vi "Output BPM.vi"(4 "error in (no error)":errorcluster, 7 "BPM (input)":dbl) -> (0 "error out":errorcluster, 3 "BPM (output)":string)   [LabVIEW 2012]
doc: "Takes the BPM input and outputs the BPM as a string after a certain number of samples, otherwise the VI returns the \"Calibrating...\" message as the filter may still be settling"
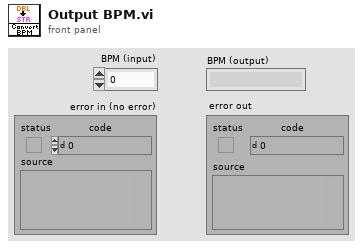
[diagram p1: front panel]
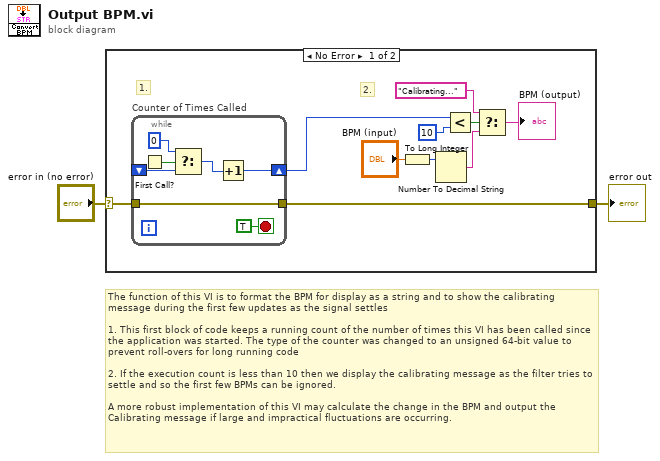
[diagram p0: block diagram]
diagram:
  # "The function of this VI is to format the BPM for display as a string and to show the calibrating message during the first few updates as the signal settles\n\n1. This first block of code keeps a running count of the number of times this VI has been called since the application was started. The type of the counter was changed to an unsigned 64-bit value to prevent roll-overs for long running code\n\n2. If the execution count is less than 10 then we display the calibrating message as the filter tries to settle and so the first few BPMs can be ignored.\n\nA more robust implementation of this VI may calculate the change in the BPM and output the Calibrating message if large and impractical fluctuations are occurring."
  n1 = case shown="No Error" "error in (no error)" {
    selector: "error in (no error)" -> [w3 w20]
    tunnel: [w12 w20] -> w2
    frame No Error {
      # "2."
      # "1."
      n2 = while "Counter of Times Called" {
        shift-right: [w18] -> w4
        shift-left: _ -> [w14]
        tunnel: w3 -> [w17]
        tunnel: [w17] -> w12
        stop <- TRUE stop-if-true
        n3 = First Call?() -> (First Call?: T/F=w16:bool)
        n4 = Select(t=u64 0, s=w16, f=w14) -> (s? t:f=w13:u64)
        n5 = Increment(x=w13) -> (x+1=w18:u64)
      }
      n6 = To Long Integer(number="BPM (input)") -> (32bit integer=w9:i32)
      n7 = Number To Decimal String(number=w9) -> (decimal integer string=w6:string)  [unwired: 1 in]
      n8 = Less?(x=w4, y=u64 10) -> (x < y?=w11:bool)
      n9 = Select(t="Calibrating...", s=w11, f=w6) -> (s? t:f=→"BPM (output)":string)
    }
    frame Error {
    }
  }
  "error out" <- w2
